vi "Test Scripts.vi"(8 "error in (no error)":errorcluster) -> (0 "error out":errorcluster)   [LabVIEW 2016]
uses:
  <vilib>/addons/_JKI Toolkits/Caraya/classes/Assert/Assert True.vi
  Source/SG/SG.lvlib
  <vilib>/addons/_JKI Toolkits/Caraya/classes/Assert/Assert.lvclass
  <vilib>/addons/_JKI Toolkits/Caraya/classes/Test/Test.lvclass
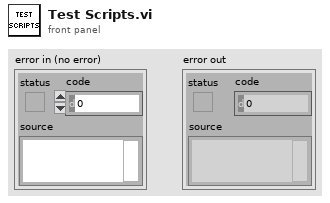
[diagram p1: front panel]
types:
  T1 = enum16{"No error on apply waveform attributes with empty script", "RDL abort function waits appropriate amount of time prior to error"}
  T2 = typedef "SG.lvlib/Waveform.ctl" = cluster{"Waveform Name":string, "Waveform":cluster{"x0":dbl, "dx":dbl, "y":csg[]}, "Signal Bandwidth (Hz)":dbl, "PAPR (dB)":dbl, "Burst Length (s)":dbl, "Sample Rate":dbl, "Burst Start Locations":i32[], "Burst Stop Locations":i32[], "Idle Duration Present?":bool, "Runtime Scaling":dbl, "Script":string}
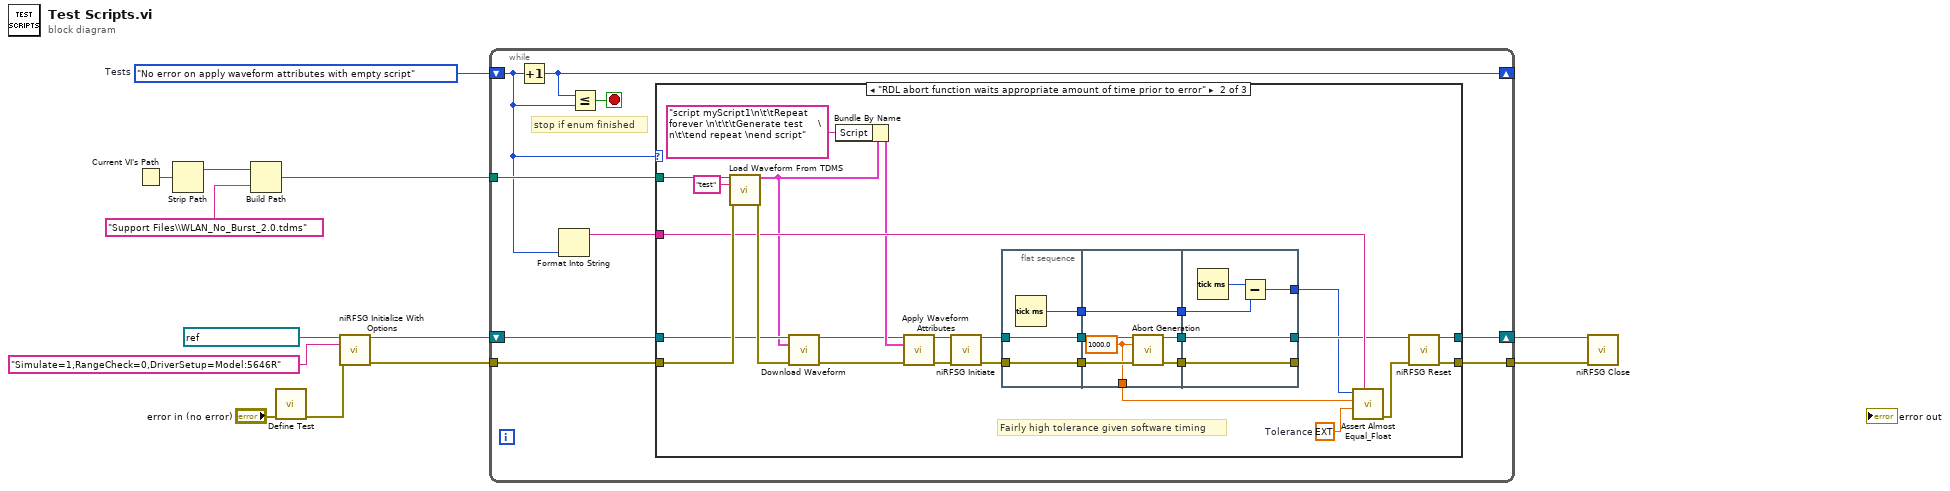
[diagram p0: block diagram]
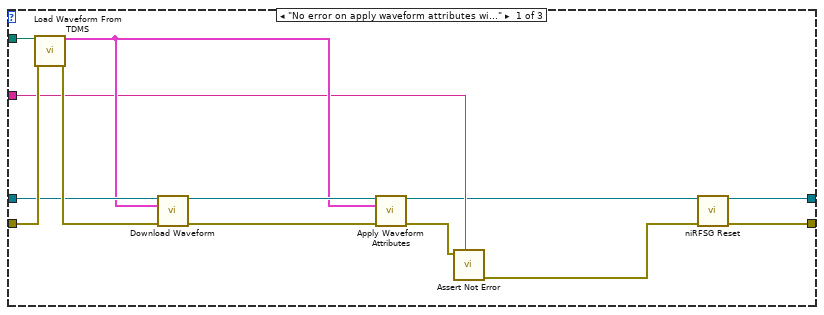
[diagram p2: hidden frame]
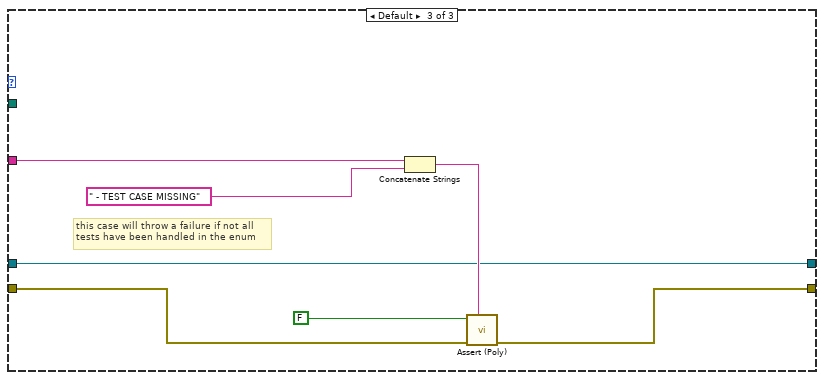
[diagram p3: hidden frame]
diagram:
  w1 = T1."No error on apply waveform attributes with empty script"  # Tests
  n1 = Current VI's Path() -> (path=w12:path)
  n2 = Strip Path(path=w12) -> (stripped path=w11:path)  [unwired: 1 out]
  n3 = Build Path(base path=w11, name or relative path="Support Files\\WLAN_No_Burst_2.0.tdms") -> (appended path=w7:path)
  n4 = call <vilib>:"Define Test.vi"("error in (no error)"="error in (no error)") -> ("error out"=w3:errorcluster)  [unwired: 10 in]
  n5 = call <instrlib>:"niRFSG Initialize With Options.vi"("resource name"=refnum<k15> "SimulatedDevice", "option string"="Simulate=1,RangeCheck=0,DriverSetup=Model:5646R", "error in"=w3) -> ("instrument handle"=w6:refnum<k15>, "error out"=w13:errorcluster)  [unwired: 11 in]
  n6 = while {
    tunnel: w7 -> [w21]
    shift-right: [w19] -> w5
    shift-left: w6 -> [w20]
    shift-right: [w17] -> _
    shift-left: w1 -> [w15]
    tunnel: w13 -> [w22]
    tunnel: [w18] -> w2
    stop <- w16 stop-if-true
    # "stop if enum finished"
    n7 = Increment(x=w15) -> (x+1=w17:T1)
    n8 = Format Into String(w15) -> (resulting string=w14:string)  [unwired: 3 in, 1 out]
    n9 = Less Or Equal?(x=w17, y=w15) -> (x <= y?=w16:bool)
    n10 = case shown="\"RDL abort function waits appropriate amount of time prior to error\"" w15 {
      tunnel: w22 -> [w35 w63 w81]
      tunnel: w21 -> [w33 w61 _]
      tunnel: w20 -> [w32 w60 w79]
      tunnel: [w23 w54 w79] -> w19
      tunnel: [w25 w55 w80] -> w18
      tunnel: w14 -> [w26 w56 w78]
      frame "No error on apply waveform attributes with empty script" {
        n11 = call "Load Waveform From TDMS.vi"("TDMS File Path"=w33, "error in (no error)"=w35) -> ("Waveform"=w29:T2, "error out"=w34:errorcluster)  [unwired: 12 in]
        n12 = call "Download Waveform.vi"("RFSG handle"=w32, "Waveform In"=w29, "error in (no error)"=w34) -> ("RFSG handle out"=w31:refnum<k15>, "error out"=w30:errorcluster)  [unwired: 11 in]
        n13 = call "Apply Waveform Attributes.vi"("RFSG Session In"=w31, "Waveform"=w29, "error in (no error)"=w30) -> ("RFSG Session Out"=w24:refnum<k15>, "error out"=w28:errorcluster)  [unwired: 11 in]
        n14 = call <vilib>:"Assert Not Error.vi"("Label"=w26, "Not Error?"=w28) -> ("error out"=w27:errorcluster)  [unwired: 9 in]
        n15 = call <instrlib>:"niRFSG Reset.vi"("instrument handle"=w24, "error in"=w27) -> ("instrument handle out"=w23:refnum<k15>, "error out"=w25:errorcluster)  [unwired: 12 in]
      }
      frame "RDL abort function waits appropriate amount of time prior to error" {
        w36 = ext 30.0  # Tolerance
        # "Fairly high tolerance given software timing"
        n16 = call "Load Waveform From TDMS.vi"("TDMS File Path"=w61, "Waveform Name (File Name)"="test", "error in (no error)"=w63) -> ("Waveform"=w51:T2, "error out"=w62:errorcluster)  [unwired: 11 in]
        n17 = call "Download Waveform.vi"("RFSG handle"=w60, "Waveform In"=w51, "error in (no error)"=w62) -> ("RFSG handle out"=w45:refnum<k15>, "error out"=w59:errorcluster)  [unwired: 11 in]
        n18 = Bundle By Name(cluster=w51, "Script"="script myScript1\n\t\tRepeat forever \n\t\t\tGenerate test     \n\t\tend repeat \nend script") -> (w50:T2)
        n19 = call "Apply Waveform Attributes.vi"("RFSG Session In"=w45, "Waveform"=w50, "error in (no error)"=w59) -> ("RFSG Session Out"=w49:refnum<k15>, "error out"=w58:errorcluster)  [unwired: 11 in]
        n20 = call <instrlib>:"niRFSG Initiate.vi"("instrument handle"=w49, "error in"=w58) -> ("instrument handle out"=w48:refnum<k15>, "error out"=w47:errorcluster)  [unwired: 12 in]
        n21 = flat-sequence {
          tunnel: w47 -> [w65]
          tunnel: w48 -> [w66]
          tunnel: [w66] -> w44
          tunnel: [w65] -> w43
          tunnel: [w64] -> w39
          tunnel: w44 -> [w72]
          tunnel: w43 -> [w71]
          tunnel: [w70] -> w42
          tunnel: [w69] -> w41
          tunnel: [w68] -> w40
          tunnel: w39 -> [w68]
          tunnel: [w67] -> w37
          tunnel: [w76] -> w46
          tunnel: [w77] -> _
          tunnel: w42 -> [w77]
          tunnel: w41 -> [w76]
          tunnel: w40 -> [w74]
          tunnel: [w73] -> w38
          frame #0 {
            n22 = Tick Count (ms)() -> (millisecond timer value=w64:u32)
          }
          frame #1 {
            w67 = 1000.0 ("Timeout (ms)")
            n23 = call "Abort Generation.vi"("RFSG handle"=w72, "Timeout (ms)"=w67, "error in (no error)"=w71) -> ("RFSG handle out"=w69:refnum<k15>, "error out"=w70:errorcluster)  [unwired: 11 in]
          }
          frame #2 {
            n24 = Tick Count (ms)() -> (millisecond timer value=w75:u32)
            n25 = Subtract(x=w75, y=w74) -> (x-y=w73:u32)
          }
        }
        n26 = call <vilib>:"Assert Almost Equal_Float.vi"("Label"=w56, "Tolerance"=w36, "Y"=w37, "X"=w38) -> ("error out"=w57:errorcluster)  [unwired: 7 in]
        n27 = call <instrlib>:"niRFSG Reset.vi"("instrument handle"=w46, "error in"=w57) -> ("instrument handle out"=w54:refnum<k15>, "error out"=w55:errorcluster)  [unwired: 12 in]
      }
      frame Default {
        # "this case will throw a failure if not all\ntests have been handled in the enum"
        n28 = Concatenate Strings(w78, " - TEST CASE MISSING" ("Label")) -> (w82:string)
        n29 = call-poly <vilib>:"Assert (Poly).vi"("Label"=w82, "error in (no error)"=w81, "True?"=FALSE) -> ("error out"=w80:errorcluster)  [unwired: 8 in]
      }
    }
  }
  n30 = call <instrlib>:"niRFSG Close.vi"("instrument handle"=w5, "error in"=w2) -> ()  [unwired: 13 in, 1 out]
